vi "Index Process Info.vi"(0 "process information":dbl[](array[numeric])) -> (14 "LabVIEW Thread Count":dbl, 15 "LabVIEW HandleCount":dbl, 16 "LabVIEW  Memory Used (MB)":dbl, 17 "Sequence Editor Thread Count":dbl, 18 "Sequence Editor  HandleCount":dbl, 19 "Sequence Editor Memory (MB)":dbl)   [LabVIEW 2016]
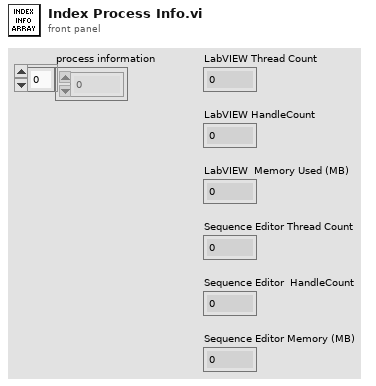
[diagram p1: front panel]
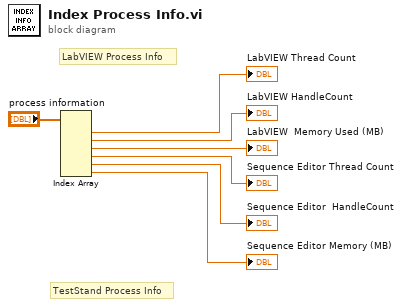
[diagram p0: block diagram]
diagram:
  # "TestStand Process Info"
  # "LabVIEW Process Info"
  n1 = Index Array(array="process information") -> (element #1=→"LabVIEW Thread Count":dbl, element #2=→"LabVIEW HandleCount":dbl, element #3=→"LabVIEW  Memory Used (MB)":dbl, element #4=→"Sequence Editor Thread Count":dbl, element #5=→"Sequence Editor  HandleCount":dbl, element #6=→"Sequence Editor Memory (MB)":dbl)  [unwired: 6 in]
